vi "Left Encoder Reset.vi"   [LabVIEW 2015]
uses:
  Support/Global Objects.vi
types:
  T1 = typedef "Encoder Info.ctl" = cluster{"EncoderDevRef":T2, "Velocity Samples":dbl[], "Velocity Index":u32}
  T2 = typedef "WPI_EncoderDevRef.ctl" = cluster{"DevStatus":errorcluster, "EncoderIndex":T3, "CounterIndex":T4, "DistancePerCount":dbl, "Decoding Type":T5}
  T3 = typedef "FPGA_EncoderIdx.ctl" = enum8{"Enc 0", "Enc 1", "Enc 2", "Enc 3", "Enc 4", "Enc 5", "Enc 6", "Enc 7", "Invalid"}
  T4 = typedef "FPGA_CounterCtrSystemIndex.ctl" = enum8{"Ctr 0", "Ctr 1", "Ctr 2", "Ctr 3", "Ctr 4", "Ctr 5", "Ctr 6", "Ctr 7", "Invalid"}
  T5 = typedef "WPI_EncoderType.ctl" = enum16{"1x", "2x", "4x"}
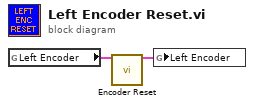
[diagram p0: block diagram]
diagram:
  n1 = global read "Global Objects.vi" "Left Encoder"() -> (w2:T1)
  n2 = call "Encoder Reset.vi"("Encoder Info"=w2) -> ("Encoder Out"=w1:T1)  [unwired: 14 in]
  n3 = global write "Global Objects.vi" "Left Encoder"(w1) -> ()
